vi "DigOP_CTRL.vi"(8 "Error In":errorcluster, 9 "Output Value":bool, 10 "Channel No":T1 items=["7"=7, "11"=11, "12"=12, "13"=13, "15"=15, "16"=16, "18"=18, "29"=29, "32"=32, "33"=33, "35"=35, "36"=36, "37"=37, "38"=38, "40"=40], 11 "LINX Resource In":T2) -> (0 "Error Out":errorcluster, 2 "Channel No":T1 items=["7"=7, "11"=11, "12"=12, "13"=13, "15"=15, "16"=16, "18"=18, "29"=29, "32"=32, "33"=33, "35"=35, "36"=36, "37"=37, "38"=38, "40"=40], 3 "LINX Resource Out":T2)   [LabVIEW 2014, in "Main.lvlib"]
uses:
  <vilib>/MakerHub/LINX/Private/Type Defs/LINX Ref.ctl
  <vilib>/MakerHub/LINX/Private/Type Defs/Platform.ctl
  <vilib>/MakerHub/LINX/Private/Type Defs/Interface.ctl
  <vilib>/MakerHub/LINX/Private/Device/Type Defs/LINX Device Config.ctl
  <vilib>/MakerHub/LINX/Private/Device/Type Defs/TCP Config.ctl
  <vilib>/MakerHub/LINX/Private/Device/Type Defs/Channels.ctl
  ValveCTRL/TypeDef/CHs_List.ctl
  <vilib>/MakerHub/LINX/Public/Peripherals/Digital/Digital Write 1 Chan.vi
  <vilib>/MakerHub/LINX/Public/Peripherals/Digital/Digital Write N Chans.vi
  <vilib>/MakerHub/LINX/Private/Local IO/LinxDigitalWrite.vi
  <vilib>/MakerHub/LINX/Public/Utilities/Check Channel.vi
  <vilib>/MakerHub/LINX/Private/Local IO/Handle Errors.vi
  <vilib>/MakerHub/LINX/Private/Utilties/Generate Error.vi
  Main.lvlib
  <vilib>/MakerHub/LINX/LMH-LINX.lvlib
  <vilib>/MakerHub/LINX/Private/Device/Device.lvlib
  ValveCTRL/ValveCTRL.lvlib
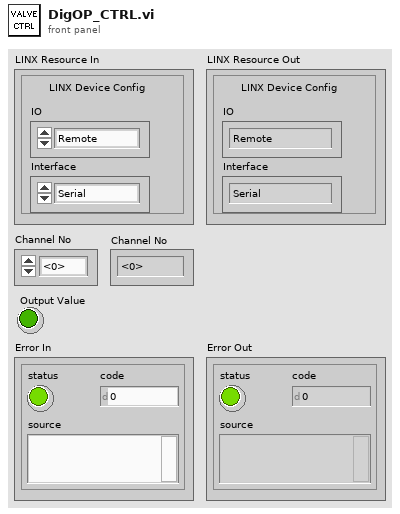
[diagram p1: front panel]
types:
  T1 = typedef "ValveCTRL.lvlib/CHs_List.ctl" = u8
  T2 = typedef "LMH-LINX.lvlib/LINX Ref.ctl" = cluster{"IO":T3, "Interface":T4, "LINX Device Config":T5}
  T3 = typedef "LMH-LINX.lvlib/Platform.ctl" = enum16{"Remote", "Local"}
  T4 = typedef "LMH-LINX.lvlib/Interface.ctl" = enum16{"Serial", "TCP"}
  T5 = typedef "LMH-LINX.lvlib/Device.lvlib/LINX Device Config.ctl" = cluster{"Interface":T4, "COM Port":refnum<visa-resource-name>, "TCP Configuration":T6, "Device Family":u8, "Device ID":u8, "Device Name":string, "TCP Ref":refnum<k5>, "Channels":T7}
  T6 = typedef "LMH-LINX.lvlib/Device.lvlib/TCP Config.ctl" = cluster{"IP Address":string, "Port":u16}
  T7 = typedef "LMH-LINX.lvlib/Channels.ctl" = cluster{"DI":u8[], "DO":u8[], "AI":u8[], "AO":u8[], "PWM":u8[], "QE":u8[], "UART":u8[], "I2C 2":u8[], "SPI":u8[], "CAN":u8[], "Servo":u8[], "AI Ref (V)":dbl, "AI Resolution (Bits)":u8, "AO Ref (V)":dbl, "AO Resolution (Bits)":u8}
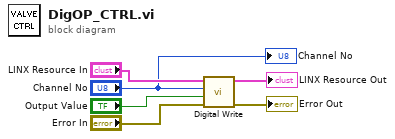
[diagram p0: block diagram]
diagram:
  n1 = call-poly <vilib>:"Digital Write.vi"("Error In"="Error In", "Output Value"="Output Value", "DO Channel"="Channel No", "LINX Resource"="LINX Resource In") -> ("Error Out"=→"Error Out":errorcluster, "LINX Resource"=→"LINX Resource Out":T2)  [unwired: 6 in]
  "Channel No" <- "Channel No"
